vi "numlock close.vi"(8 "error in (no error)":errorcluster, 11 "logger":T1) -> (0 "error out":errorcluster, 3 "file path out":path)   [LabVIEW 2019]
doc: "Closes the tdms file and returns the path"
uses:
  numlock.ctl
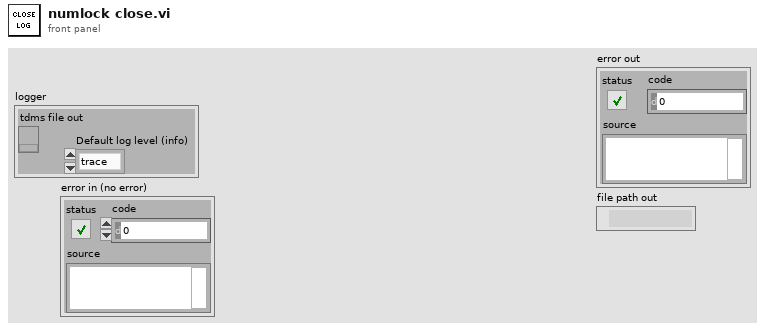
[diagram p1: front panel]
types:
  T1 = typedef "numlock.ctl" = cluster{"tdms file out":refnum<k34>, "Default log level (info)":enum16{"trace", "debug", "info", "warn", "error"}}
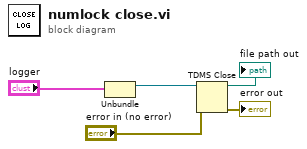
[diagram p0: block diagram]
diagram:
  n1 = Unbundle("logger") -> ("tdms file out"=w5:refnum<k34>)  [unwired: 1 out]
  n2 = TDMS Close(8:"error in (no error)", 11:w5) -> (0:→"error out":errorcluster, 3:→"file path out":path)
